vi "From BananaPips.vi"(11 "Pips.TestResults":refnum<class "Pips.TestResults.lvclass">) -> (2 "Test Result":refnum<class "Test Result.lvclass">)   [LabVIEW 2021, in "Banana.Caraya.lvlib" / "Pips.TestResults.lvclass"]
uses:
  Pips.TestResults.lvclass
  Pips.TestResults.lvclass/Pips.TestResults.ctl
  <vilib>/addons/_JKI Toolkits/Caraya/classes/Test Result/Test Result.lvclass
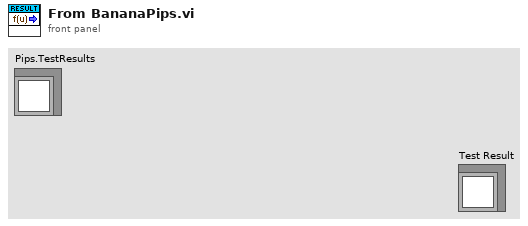
[diagram p1: front panel]
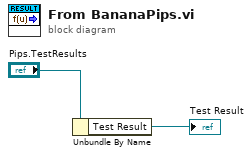
[diagram p0: block diagram]
diagram:
  n1 = Unbundle By Name("Pips.TestResults") -> ("Test Result"=→"Test Result":refnum<class "Test Result.lvclass">)
